vi "4_1_MNIST_Drawing_Interface(CPU).vi"() -> ()   [LabVIEW 2020]
doc: "This is a support VI for MNIST_deploy(RT).vi for handwritten digit intensity map generation on PC and transfer onto RT target.\nRequirements: Deep Learning Toolkit for LabVIEW."
panel:
  out "Pen Attributes":T1={"Width"=35, "Style"=enum."Solid"}
  out "Draw Digit (280x280px)":picture
  in  "Pen Color":u32(colorbox)=197379
  in  "Clear":bool
  in  "Pen Width":u16=24
  in  "Stop Test":bool
  out "Image (28x28px)":sgl[][](graph)=[[-1.0, -1.0, -1.0, -1.0, -1.0, -1.0, -1.0, -1.0, -1.0, -1.0, -1.0, -1.0, -1.0, -1.0, -1.0, -1.0, -1.0, -1.0, -1.0, -1.0, -1.0, -1.0, -1.0, -1.0, -1.0, -1.0, -1.0, -1.0], [-1.0, -1.0, -1.0, -1.0, -1.0, -1.0, -1.0, -1.0, -1.0, -1.0, -1.0, -1.0, -1.0, -1.0, -1.0, -1.0, -1.0, -1.0, -1.0, -1.0, -1.0, -1.0, -1.0, -1.0, -1.0, -1.0, -1.0, -1.0], [-1.0, -1.0, -1.0, -1.0, -1.0, -1.0, -1.0, -1.0, -1.0, -1.0, -1.0, -1.0, -1.0, -1.0, -1.0, -1.0, -1.0, -1.0, -1.0, -1.0, -1.0, -1.0, -1.0, -1.0, -1.0, -1.0, -1.0, -1.0], [-1.0, -1.0, -1.0, -1.0, -1.0, -1.0, -1.0, -1.0, -1.0, -1.0, -1.0, -1.0, -1.0, -1.0, -1.0, -1.0, -1.0, -1.0, -1.0, -1.0, -1.0, -1.0, -1.0, -1.0, -1.0, -1.0, -1.0, -1.0], [-1.0, -1.0, -1.0, -1.0, -1.0, -1.0, -1.0, -1.0, -1.0, -1.0, -1.0, -1.0, -1.0, -1.0, -1.0, -1.0, -1.0, -1.0, -1.0, -1.0, -1.0, -1.0, -1.0, -1.0, -1.0, -1.0, -1.0, -1.0], [-1.0, -1.0, -1.0, -1.0, -1.0, -1.0, -1.0, -1.0, -1.0, -1.0, -1.0, -1.0, -1.0, -1.0, -1.0, -1.0, -1.0, -1.0, -1.0, -1.0, -1.0, -1.0, -1.0, -1.0, -1.0, -1.0, -1.0, -1.0], [-1.0, -1.0, -1.0, -1.0, -1.0, -1.0, -1.0, -1.0, -1.0, -1.0, -1.0, -1.0, -1.0, -1.0, -1.0, -1.0, -1.0, -1.0, -1.0, -1.0, -1.0, -1.0, -1.0, -1.0, -1.0, -1.0, -1.0, -1.0], [-1.0, -1.0, -1.0, -1.0, -1.0, -1.0, -1.0, -1.0, -1.0, -1.0, -1.0, -1.0, -1.0, -1.0, -1.0, -1.0, -1.0, -1.0, -1.0, -1.0, -1.0, -1.0, -1.0, -1.0, -1.0, -1.0, -1.0, -1.0], [-1.0, -1.0, -1.0, -1.0, -1.0, -1.0, -1.0, -1.0, -1.0, -1.0, -1.0, -1.0, -1.0, -1.0, -1.0, -1.0, -1.0, -1.0, -1.0, -1.0, -1.0, -1.0, -1.0, -1.0, -1.0, -1.0, -1.0, -1.0], [-1.0, -1.0, -1.0, -1.0, -1.0, -1.0, -1.0, -1.0, -1.0, -1.0, -1.0, -1.0, -1.0, -1.0, -1.0, -1.0, -1.0, -1.0, -1.0, -1.0, -1.0, -1.0, -1.0, -1.0, -1.0, -1.0, -1.0, -1.0], [-1.0, -1.0, -1.0, -1.0, -1.0, -1.0, -1.0, -1.0, -1.0, -1.0, -1.0, -1.0, -1.0, -1.0, -1.0, -1.0, -1.0, -1.0, -1.0, -1.0, -1.0, -1.0, -1.0, -1.0, -1.0, -1.0, -1.0, -1.0], [-1.0, -1.0, -1.0, -1.0, -1.0, -1.0, -1.0, -1.0, -1.0, -1.0, -1.0, -1.0, -1.0, -1.0, -1.0, -1.0, -1.0, -1.0, -1.0, -1.0, -1.0, -1.0, -1.0, -1.0, -1.0, -1.0, -1.0, -1.0], [-1.0, -1.0, -1.0, -1.0, -1.0, -1.0, -1.0, -1.0, -1.0, -1.0, -1.0, -1.0, -1.0, -1.0, -1.0, -1.0, -1.0, -1.0, -1.0, -1.0, -1.0, -1.0, -1.0, -1.0, -1.0, -1.0, -1.0, -1.0], [-1.0, -1.0, -1.0, -1.0, -1.0, -1.0, -1.0, -1.0, -1.0, -1.0, -1.0, -1.0, -1.0, -1.0, -1.0, -1.0, -1.0, -1.0, -1.0, -1.0, -1.0, -1.0, -1.0, -1.0, -1.0, -1.0, -1.0, -1.0], [-1.0, -1.0, -1.0, -1.0, -1.0, -1.0, -1.0, -1.0, -1.0, -1.0, -1.0, -1.0, -1.0, -1.0, -1.0, -1.0, -1.0, -1.0, -1.0, -1.0, -1.0, -1.0, -1.0, -1.0, -1.0, -1.0, -1.0, -1.0], [-1.0, -1.0, -1.0, -1.0, -1.0, -1.0, -1.0, -1.0, -1.0, -1.0, -1.0, -1.0, -1.0, -1.0, -1.0, -1.0, -1.0, -1.0, -1.0, -1.0, -1.0, -1.0, -1.0, -1.0, -1.0, -1.0, -1.0, -1.0], [-1.0, -1.0, -1.0, -1.0, -1.0, -1.0, -1.0, -1.0, -1.0, -1.0, -1.0, -1.0, -1.0, -1.0, -1.0, -1.0, -1.0, -1.0, -1.0, -1.0, -1.0, -1.0, -1.0, -1.0, -1.0, -1.0, -1.0, -1.0], [-1.0, -1.0, -1.0, -1.0, -1.0, -1.0, -1.0, -1.0, -1.0, -1.0, -1.0, -1.0, -1.0, -1.0, -1.0, -1.0, -1.0, -1.0, -1.0, -1.0, -1.0, -1.0, -1.0, -1.0, -1.0, -1.0, -1.0, -1.0], [-1.0, -1.0, -1.0, -1.0, -1.0, -1.0, -1.0, -1.0, -1.0, -1.0, -1.0, -1.0, -1.0, -1.0, -1.0, -1.0, -1.0, -1.0, -1.0, -1.0, -1.0, -1.0, -1.0, -1.0, -1.0, -1.0, -1.0, -1.0], [-1.0, -1.0, -1.0, -1.0, -1.0, -1.0, -1.0, -1.0, -1.0, -1.0, -1.0, -1.0, -1.0, -1.0, -1.0, -1.0, -1.0, -1.0, -1.0, -1.0, -1.0, -1.0, -1.0, -1.0, -1.0, -1.0, -1.0, -1.0], [-1.0, -1.0, -1.0, -1.0, -1.0, -1.0, -1.0, -1.0, -1.0, -1.0, -1.0, -1.0, -1.0, -1.0, -1.0, -1.0, -1.0, -1.0, -1.0, -1.0, -1.0, -1.0, -1.0, -1.0, -1.0, -1.0, -1.0, -1.0], [-1.0, -1.0, -1.0, -1.0, -1.0, -1.0, -1.0, -1.0, -1.0, -1.0, -1.0, -1.0, -1.0, -1.0, -1.0, -1.0, -1.0, -1.0, -1.0, -1.0, -1.0, -1.0, -1.0, -1.0, -1.0, -1.0, -1.0, -1.0], [-1.0, -1.0, -1.0, -1.0, -1.0, -1.0, -1.0, -1.0, -1.0, -1.0, -1.0, -1.0, -1.0, -1.0, -1.0, -1.0, -1.0, -1.0, -1.0, -1.0, -1.0, -1.0, -1.0, -1.0, -1.0, -1.0, -1.0, -1.0], [-1.0, -1.0, -1.0, -1.0, -1.0, -1.0, -1.0, -1.0, -1.0, -1.0, -1.0, -1.0, -1.0, -1.0, -1.0, -1.0, -1.0, -1.0, -1.0, -1.0, -1.0, -1.0, -1.0, -1.0, -1.0, -1.0, -1.0, -1.0], [-1.0, -1.0, -1.0, -1.0, -1.0, -1.0, -1.0, -1.0, -1.0, -1.0, -1.0, -1.0, -1.0, -1.0, -1.0, -1.0, -1.0, -1.0, -1.0, -1.0, -1.0, -1.0, -1.0, -1.0, -1.0, -1.0, -1.0, -1.0], [-1.0, -1.0, -1.0, -1.0, -1.0, -1.0, -1.0, -1.0, -1.0, -1.0, -1.0, -1.0, -1.0, -1.0, -1.0, -1.0, -1.0, -1.0, -1.0, -1.0, -1.0, -1.0, -1.0, -1.0, -1.0, -1.0, -1.0, -1.0], [-1.0, -1.0, -1.0, -1.0, -1.0, -1.0, -1.0, -1.0, -1.0, -1.0, -1.0, -1.0, -1.0, -1.0, -1.0, -1.0, -1.0, -1.0, -1.0, -1.0, -1.0, -1.0, -1.0, -1.0, -1.0, -1.0, -1.0, -1.0], [-1.0, -1.0, -1.0, -1.0, -1.0, -1.0, -1.0, -1.0, -1.0, -1.0, -1.0, -1.0, -1.0, -1.0, -1.0, -1.0, -1.0, -1.0, -1.0, -1.0, -1.0, -1.0, -1.0, -1.0, -1.0, -1.0, -1.0, -1.0]]
  # "Overview: This is a support VI for MNIST_deploy(RT).vi for handwritten digit intensity map generation on PC and transfer onto RT target.\nInstructions:\n1. Run the VI.\n2. Draw a digit on the \"Draw Digit (280x280 px)\" interface.\n3. Right click on \"image (28x28px)\" and select \"Copy Data\" (copy the content of 2D array into clipboard).\n4. Go to 4_2_MNIST_Inference(CPU)(RT).vi or 4_3_MNIST_Inference(FPGA)(RT).vi and paste the data from clipboard onto \"Image (28x28px)\" interface. \n\nMore Examples:  https://github.com/ngenehub/deepltk_examples"
  # "Down sampled Copy"
  # "High resolution drawing interface"
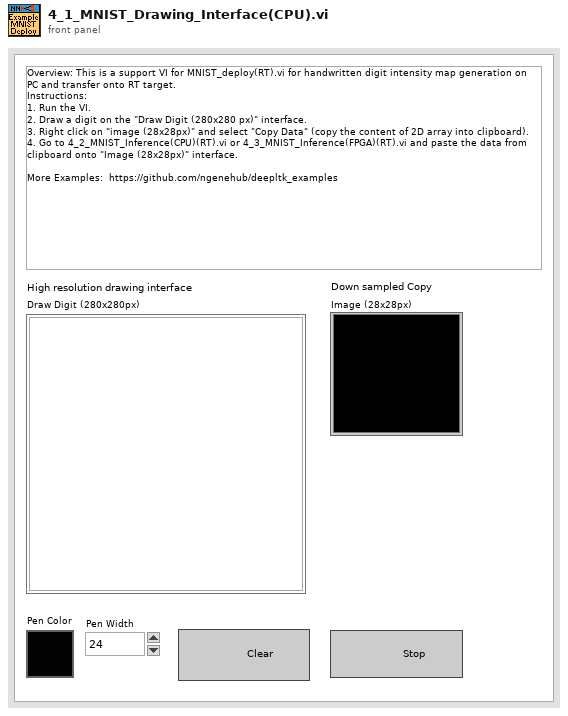
[diagram p1: front panel]
types:
  T1 = cluster{"Width":u16, "Style":enum32{"Solid", "Dash", "Dot", "DashDot", "DashDotDot"}}
  T2 = cluster{"left":i16, "top":i16, "right":i16, "bottom":i16}
  T3 = typedef "LVMouseTypeDef.ctl" = cluster{"Mouse Position":cluster{"X":i32, "Y":i32}, "Mouse Modifiers":cluster{"Button Down":bool, "Shift Mod":bool, "Menu Mod":bool, "Option Mod":bool}}
  T4 = typedef "imagedata.ctl" = cluster{"image type":i32, "image depth":i32, "image":u8[], "mask":u8[], "colors":u32[], "Rectangle":cluster{"left":i16, "top":i16, "right":i16, "bottom":i16}}
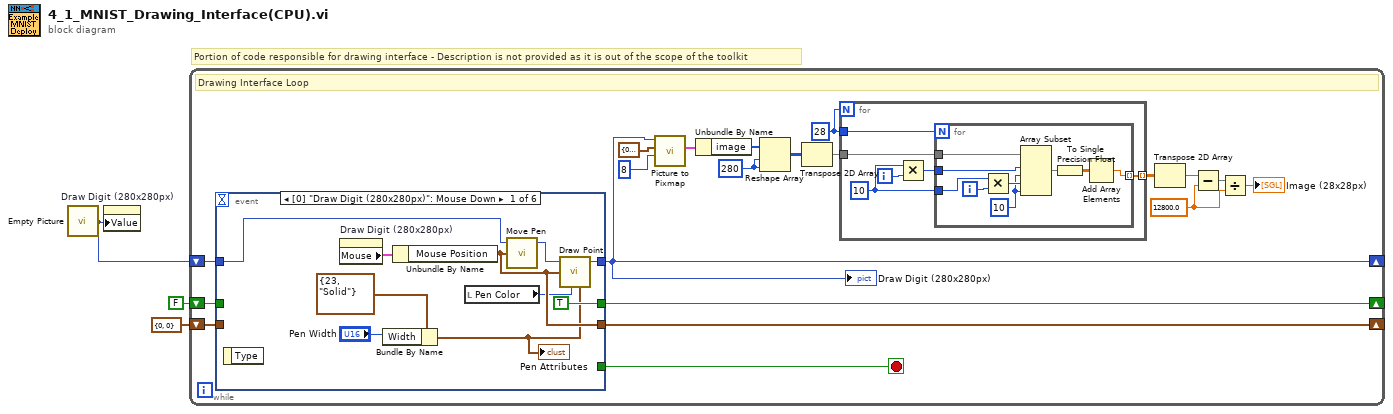
[diagram p0: block diagram]
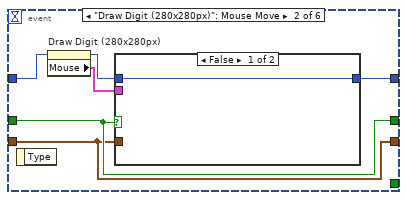
[diagram p2: hidden frame]
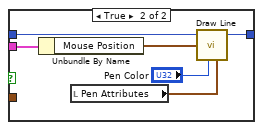
[diagram p3: hidden frame]
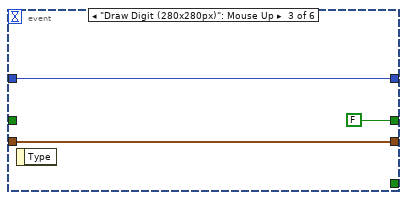
[diagram p4: hidden frame]
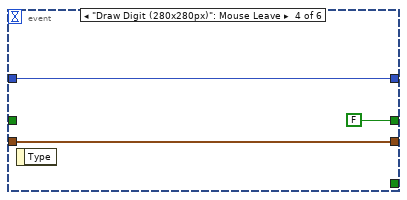
[diagram p5: hidden frame]
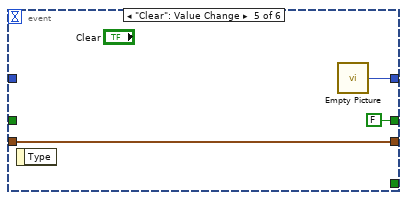
[diagram p6: hidden frame]
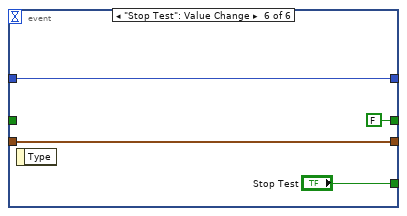
[diagram p7: hidden frame]
diagram:
  # "Portion of code responsible for drawing interface - Description is not provided as it is out of the scope of the toolkit"
  n1 = call "Empty Picture"() -> ("empty picture"=w3:picture)
  n2 = property on="Draw Digit (280x280px)" class="Pict"("Value"=w3) -> ()  [unwired: 2 in, 2 out]
  n3 = while {
    shift-right: [w18] -> _
    shift-left: w3 -> [w23]
    shift-right: [w21] -> _
    shift-left: FALSE -> [w22]
    shift-right: [w19] -> _
    shift-left: cluster{"X":i32, "Y":i32} {"X"=0, "Y"=0} ("Mouse Position") -> [w20]
    stop <- w10 stop-if-true
    w7 = sgl 12800.0 ("dimension size")
    w11 = 280 ("dimension size")
    w13 = 28
    # "Drawing Interface Loop"
    n4 = event shown="[0] \"Draw Digit (280x280px)\": Mouse Down" {
      selector: _ -> [_ _ _ _ _ _]
      dyn-events: _ -> [_ _ _ _ _ _]
      timeout: _ -> [_ _ _ _ _ _]
      tunnel: [_ _ _ _ _ "Stop Test"] -> w10
      tunnel: [w45 w52 w63 w66 w69 w72] -> w18
      tunnel: w23 -> [w47 w51 w63 w66 _ w72]
      tunnel: w22 -> [_ w50 _ _ _ _]
      tunnel: [TRUE w50 FALSE FALSE FALSE FALSE] -> w21
      tunnel: w20 -> [_ w49 w61 w65 w68 w71]
      tunnel: [w43 w49 w61 w65 w68 w71] -> w19
      event "Draw Digit (280x280px)": Mouse Down {
        # "Set the pen position, and draw an initial point or line."
        n5 = event-data() -> ()  [unwired: 1 in, 1 out]
        n6 = property on="Draw Digit (280x280px)" class="Pict"() -> ("Mouse"=w48:T3)  [unwired: 2 in, 2 out]
        n7 = Bundle By Name(cluster=T1 {"Width"=23, "Style"=enum."Solid"} ("Pen Attributes"), "Width"="Pen Width") -> (w39:T1)
        "Pen Attributes" <- w39
        n8 = Unbundle By Name(w48) -> ("Mouse Position"=w43:cluster{"X":i32, "Y":i32})
        n9 = local read "Pen Color"() -> (w42:u32)
        n10 = call <vilib>:"Move Pen.vi"("new position"=w43, "picture"=w47) -> ("new picture"=w46:picture)  [unwired: 3 in]
        n11 = call <vilib>:"Draw Point.vi"("picture"=w46, "point(x,y)"=w43, "color(black)"=w42, "pen"=w39) -> ("new picture"=w45:picture)  [unwired: 5 in]
      }
      event "Draw Digit (280x280px)": Mouse Move {
        # "Only draw if a Mouse Down event has occurred, but not a Mouse Up. Then, determine if the user is Drawing a point, a line, or selecting a subset and perform those operations in the case structure."
        n12 = event-data() -> ()  [unwired: 1 in, 1 out]
        n13 = property on="Draw Digit (280x280px)" class="Pict"() -> ("Mouse"=w53:T3)  [unwired: 2 in, 2 out]
        n14 = case shown="False" w50 {
          tunnel: w51 -> [w54 w60]
          tunnel: w53 -> [_ w59]
          tunnel: [w54 w57] -> w52
          tunnel: w49 -> [_ _]
          frame False {
          }
          frame True {
            n15 = Unbundle By Name(w59) -> ("Mouse Position"=w58:cluster{"X":i32, "Y":i32})
            n16 = local read "Pen Attributes"() -> (w56:T1)
            n17 = call <vilib>:"Draw Line.vi"("picture"=w60, "end point"=w58, "color(black)"="Pen Color", "pen"=w56) -> ("new picture"=w57:picture)  [unwired: 5 in]
          }
        }
      }
      event "Draw Digit (280x280px)": Mouse Up {
        # "When the user is finished drawing, we complete the operation. The only operation that we need to complete the Select Subset operation."
        n18 = event-data() -> ()  [unwired: 1 in, 1 out]
      }
      event "Draw Digit (280x280px)": Mouse Leave {
        # "Change to the default cursor when the mouse leaves the picture."
        n19 = event-data() -> ()  [unwired: 1 in, 1 out]
      }
      event "Clear": Value Change {
        # "Erase the picture."
        n20 = event-data() -> ()  [unwired: 1 in, 1 out]
        n21 = call "Empty Picture"() -> ("empty picture"=w69:picture)
      }
      event "Stop Test": Value Change {
        # "Stop the VI."
        n22 = event-data() -> ()  [unwired: 1 in, 1 out]
      }
    }
    "Draw Digit (280x280px)" <- w18
    n23 = call <vilib>:"Picture to Pixmap.vi"("depth"=8, "rect"=T2 {"left"=0, "top"=0, "right"=280, "bottom"=280}, "picture"=w18) -> ("image data"=w17:T4)  [unwired: 7 in, 1 out]
    n24 = Unbundle By Name(w17) -> ("image"=w16:u8[])
    n25 = Reshape Array(w16, w11, w11) -> (w15:u8[][])
    n26 = Transpose 2D Array(2D array=w15) -> (transposed array=w14:u8[][])
    n27 = for {
      N: w13 -> [_]
      tunnel: w14 -> [w29]
      tunnel: w13 -> [w28]
      tunnel: [w24] -> w12 mode=indexing
      i -> [w27]
      w25 = 10 ("x")
      n28 = Multiply(x=w25, y=w27) -> (x*y=w26:i32)
      n29 = for {
        N: w28 -> [_]
        tunnel: w29 -> [w38]
        tunnel: w26 -> [w37]
        tunnel: w25 -> [w34]
        tunnel: [w30] -> w24 mode=indexing
        i -> [w36]
        w33 = 10 ("length")
        n30 = Multiply(x=w34, y=w36) -> (x*y=w35:i32)
        n31 = Array Subset(array=w38, index (row)=w37, length (row)=w33, index (col)=w35, length (col)=w33) -> (w32:u8[][])
        n32 = To Single Precision Float(number=w32) -> (single precision float=w31:sgl[][])
        n33 = Add Array Elements(numeric array=w31) -> (sum=w30:sgl)
      }
    }
    n34 = Transpose 2D Array(2D array=w12) -> (transposed array=w8:sgl[][])
    n35 = Subtract(x=w8, y=w7) -> (x-y=w9:sgl[][])
    n36 = Divide(x=w9, y=w7) -> (x/y=→"Image (28x28px)":sgl[][])
  }
